vi "GUI.Initialization.vi"(8 "error in (no error)":errorcluster, 11 "pathToMainVI":path) -> (0 "error out":errorcluster)   [LabVIEW 2019]
uses:
  Control Reference/State.ctl
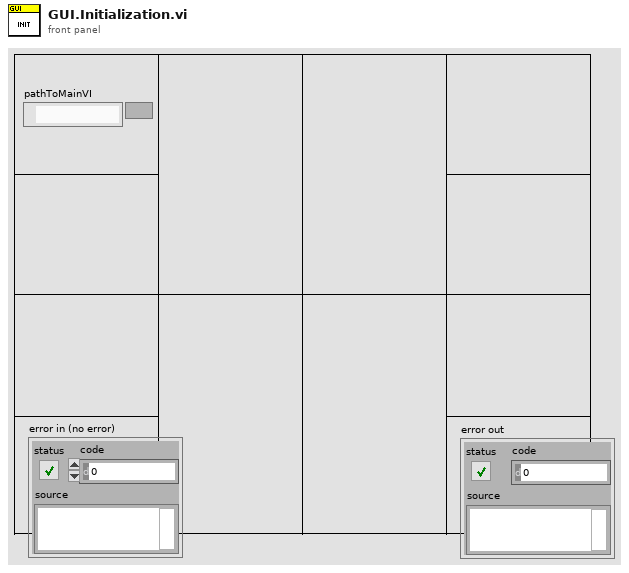
[diagram p1: front panel]
types:
  T1 = typedef "State.ctl" = enum16{"setReferences", "getReference", "closeReferences"}
  T2 = enum8{"Enabled", "Disabled", "Disabled and Grayed Out"}
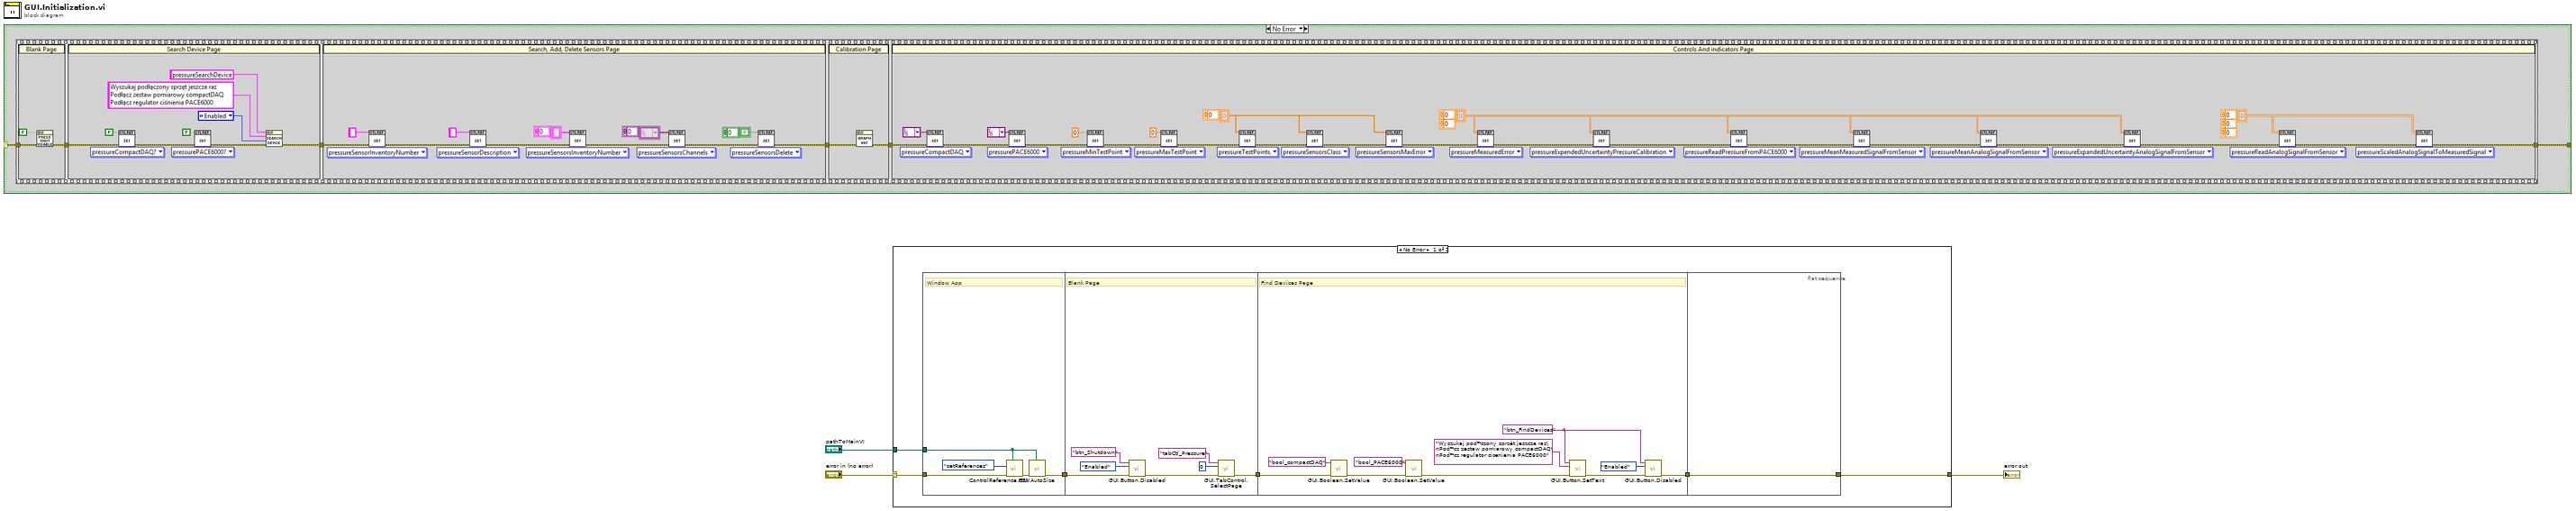
[diagram p0: block diagram]
diagram:
  n1 = case shown="No Error" "error in (no error)" {
    selector: "error in (no error)" -> [w9 w33]
    tunnel: [w5 w33] -> w1
    tunnel: "pathToMainVI" -> [w8 _]
    frame No Error {
      n2 = flat-sequence {
        tunnel: w9 -> [w11]
        tunnel: w8 -> [w10]
        tunnel: [w12] -> w7
        tunnel: w7 -> [w19]
        tunnel: [w15] -> w6
        tunnel: w6 -> [w28]
        tunnel: [w24] -> w4
        tunnel: [w32] -> w5
        tunnel: w4 -> [w32]
        frame #0 {
          # "Window App"
          n3 = call "ControlReference.FGV.vi"("pathToMainVI"=w10, "error in (no error)"=w11, "state (getReference)"=State."setReferences") -> ("error out"=w13:errorcluster)  [unwired: 7 in, 1 out]
          n4 = call "GUI.AutoSize.vi"("pathToMainVI in"=w10, "error in (no error)"=w13) -> ("error out"=w12:errorcluster)  [unwired: 9 in]
        }
        frame #1 {
          # "Blank Page"
          n5 = call "GUI.Button.Disabled.vi"("error in (no error)"=w19, "buttonDisabled"=T2."Enabled" ("Disabled"), "buttonName"="btn_Shutdown") -> ("error out"=w16:errorcluster)  [unwired: 8 in]
          n6 = call "GUI.TabControl.SelectPage.vi"("error in (no error)"=w16, "pageNumber"=0, "tabControlName"="tabCtl_Pressure" ("buttonName")) -> ("error out"=w15:errorcluster)  [unwired: 8 in]
        }
        frame #2 {
          w26 = "btn_FindDevices" ("buttonName")
          # "Find Devices Page"
          n7 = call "GUI.Boolean.SetValue.vi"("error in (no error)"=w28, "booleanName"="bool_compactDAQ") -> ("error out"=w31:errorcluster)  [unwired: 9 in]
          n8 = call "GUI.Boolean.SetValue.vi"("error in (no error)"=w31, "booleanName"="bool_PACE6000") -> ("error out"=w27:errorcluster)  [unwired: 9 in]
          n9 = call "GUI.Button.SetText.vi"("error in (no error)"=w27, "buttonText"="Wyszukaj pod³¹czony sprzêt jeszcze raz\nPod³¹cz zestaw pomiarowy compactDAQ\nPod³¹cz regulator ciœnienia PACE6000" ("controlBoolText"), "buttonName"=w26) -> ("error out"=w25:errorcluster)  [unwired: 8 in]
          n10 = call "GUI.Button.Disabled.vi"("error in (no error)"=w25, "buttonDisabled"=T2."Enabled", "buttonName"=w26) -> ("error out"=w24:errorcluster)  [unwired: 8 in]
        }
        frame #3 {
        }
      }
    }
    frame Error {
    }
  }
  "error out" <- w1
